vi "Convert Storage Class String to Enum.vi"(11 "Storage Class String":string) -> (3 "Storage Class":T1)   [LabVIEW 2015, in "NI_AWS_S3.lvlib"]
doc: "Convert the Storage Class represented as a String to the Enum typedef representation."
uses:
  NI_AWS_S3.lvlib
  Storage Class.ctl
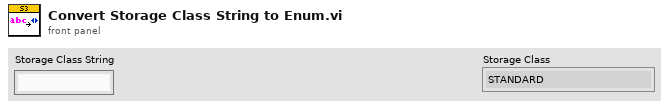
[diagram p1: front panel]
types:
  T1 = typedef "NI_AWS_S3.lvlib/Storage Class.ctl" = enum16{"STANDARD", "REDUCED_REDUNDANCY"}
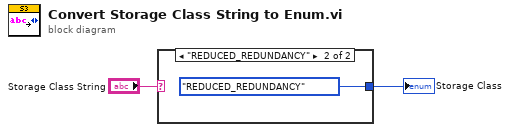
[diagram p0: block diagram]
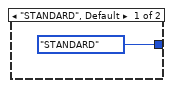
[diagram p2: hidden frame]
diagram:
  n1 = case shown="\"REDUCED_REDUNDANCY\"" "Storage Class String" {
    tunnel: [Storage_Class."STANDARD" ("Storage Class") Storage_Class."REDUCED_REDUNDANCY" ("Storage Class")] -> w1
    frame "STANDARD", Default {
    }
    frame "REDUCED_REDUNDANCY" {
    }
  }
  "Storage Class" <- w1
